vi "Get Flow Rate.vi"(8 "error in (no error)":errorcluster, 11 "Mass Flow Controller in":refnum<class "Mass Flow Controller.lvclass">) -> (0 "error out":errorcluster, 1 "Flow Rate Units":T1, 2 "Flow Rate":dbl, 3 "Mass Flow Controller out":refnum<class "Mass Flow Controller.lvclass">)   [LabVIEW 2011, in "Mass Flow Controller.lvclass"]
uses:
  Mass Flow Controller.lvclass
  Flow Rate Units.ctl
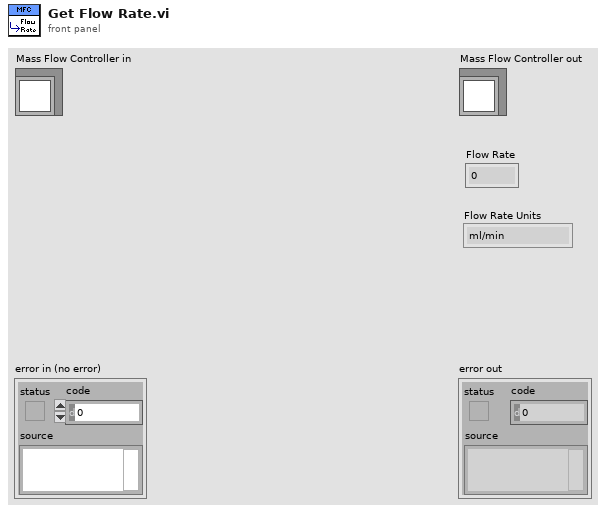
[diagram p1: front panel]
types:
  T1 = typedef "Mass Flow Controller.lvclass/Flow Rate Units.ctl" = enum16{"ml/min"}
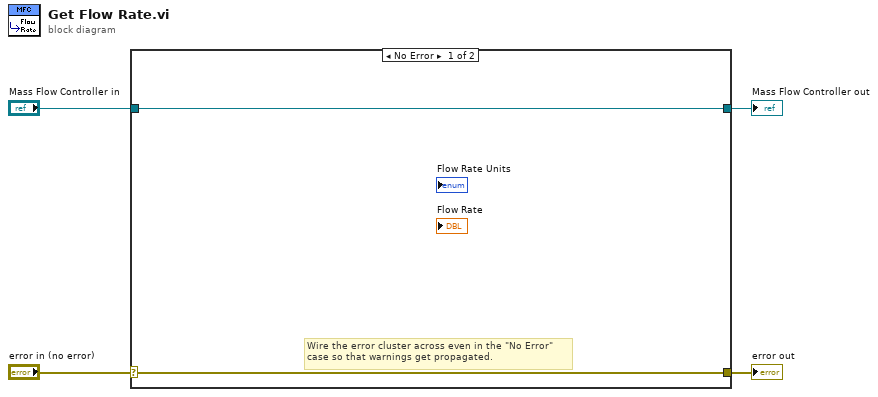
[diagram p0: block diagram]
diagram:
  n1 = case shown="No Error" "error in (no error)" {
    selector: "error in (no error)" -> [w5 w8]
    tunnel: [w5 w8] -> w3
    tunnel: [w6 w7] -> w1
    tunnel: "Mass Flow Controller in" -> [w6 w7]
    frame No Error {
      # "Wire the error cluster across even in the \"No Error\"\ncase so that warnings get propagated."
    }
    frame Error {
    }
  }
  "error out" <- w3
  "Mass Flow Controller out" <- w1
